vi "Apply LSS to GObject.vi"(8 "Error in":errorcluster, 10 "Style Sheet":string, 11 "Gen Refnum":refnum<vi>) -> (0 "Error out":errorcluster)   [LabVIEW 2019, in "LSS.lvlib"]
doc: "Parses the text from the style sheet input to find relevent properties which apply to the Gen Refnum input, then applies these properties to that control.\n\n<b>Inputs:</b>\n<b>Gen Refnum</b> - Generic reference to front panel element which will be modified by this VI.\n<b>Style Sheet</b> - Text style sheet which will be applied to the front panel element.\n<b>Error In</b> - Standard Error in terminal.\n\n<b>Outputs</b>\n<b>Error Out</b> - Standard Error Out terminal."
uses:
  LSS.lvlib
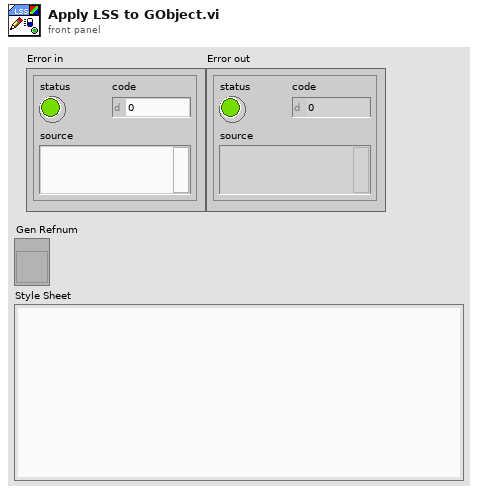
[diagram p1: front panel]
types:
  T1 = typedef "LSS.lvlib/Style.ctl" = cluster{"Specifier":string, "Properties":cluster{"Property":string, "Value":string}[]}
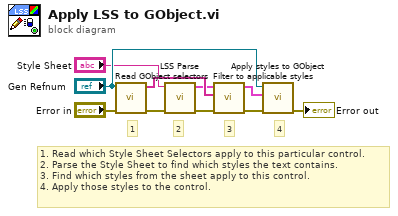
[diagram p0: block diagram]
diagram:
  # "1. Read which Style Sheet Selectors apply to this particular control.\n2. Parse the Style Sheet to find which styles the text contains.\n3. Find which styles from the sheet apply to this control.\n4. Apply those styles to the control."
  # "4"
  # "3"
  # "2"
  # "1"
  n1 = call "Read GObject selectors.vi"("Error in"="Error in", "Generic In"="Gen Refnum") -> ("Error out"=w2:errorcluster, "Selectors"=w10:string[])  [unwired: 8 in]
  n2 = call "LSS Parse.vi"("Error in"=w2, "Style Sheet"="Style Sheet") -> ("Error out"=w1:errorcluster, "LSS Styles"=w9:T1[])  [unwired: 8 in]
  n3 = call "Filter to applicable styles.vi"("Error in"=w1, "Selectors"=w10, "LSS styles"=w9) -> ("Error out"=w3:errorcluster, "Applicable styles"=w8:T1[])  [unwired: 7 in]
  n4 = call "Apply styles to GObject.vi"("Error in"=w3, "Style Sheet"=w8, "Gen Refnum"="Gen Refnum") -> ("Error out"=→"Error out":errorcluster)  [unwired: 8 in]
